vi "Calib_Ch_setup.vi"(1 "Preston tube diammeter in mm":dbl, 2 "Ch & spans":T1(array[cluster])=[{"high limit (10V)"=5.0, "low limit (-10V)"=3.0, "Ch No"=1, "Var name"="Cross wire 1"}, {"high limit (10V)"=5.0, "low limit (-10V)"=3.0, "Ch No"=2, "Var name"="Cross wire 2"}] {"Ch No" min=0 max=7; "low limit (-10V)" min=-10 max=10 format="%.3f"; "high limit (10V)" min=-10 max=10 format="%.3f"}, 3 "Calib filename":path) -> (0 "Output string":string)   [LabVIEW 2010]
panel:
  out "length":i32
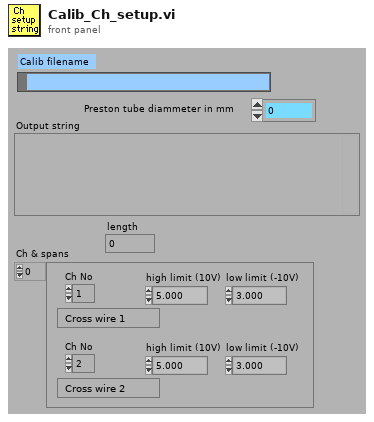
[diagram p1: front panel]
types:
  T1 = cluster{"high limit (10V)":sgl, "low limit (-10V)":sgl, "Ch No":i16, "Var name":string}[]
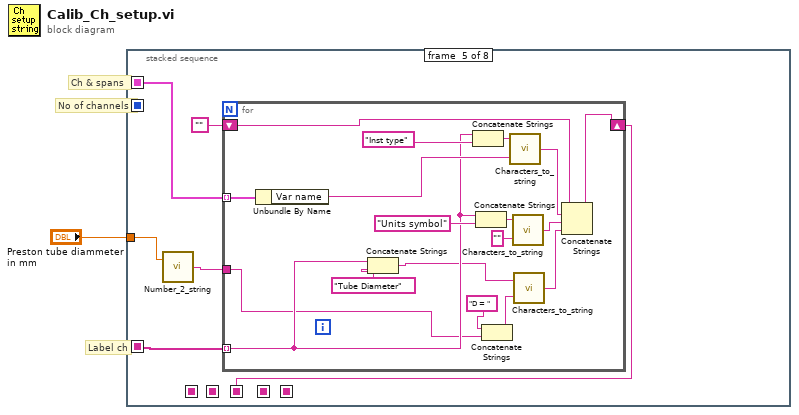
[diagram p0: block diagram]
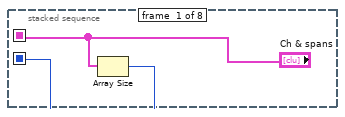
[diagram p2: hidden frame]
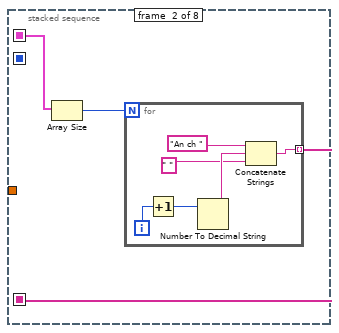
[diagram p3: hidden frame]
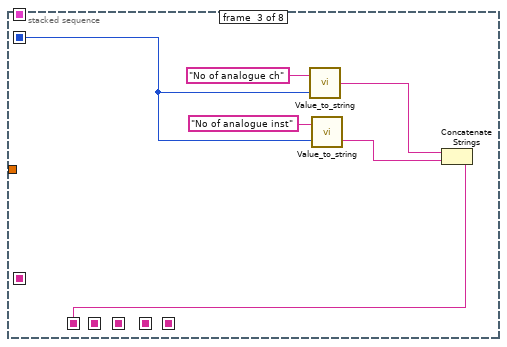
[diagram p4: hidden frame]
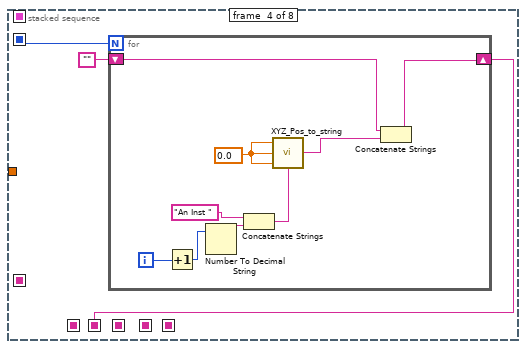
[diagram p5: hidden frame]
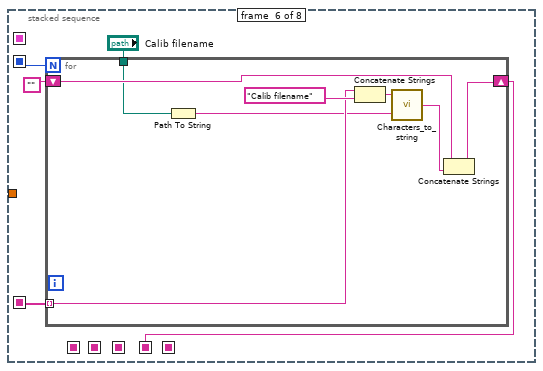
[diagram p6: hidden frame]
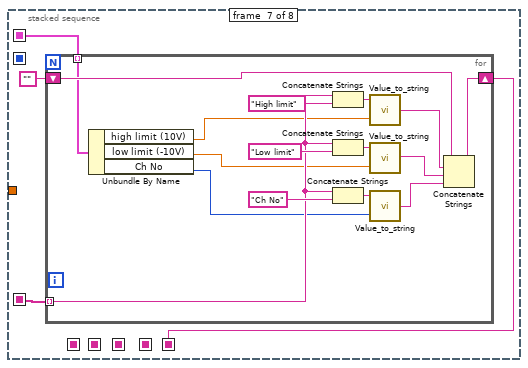
[diagram p7: hidden frame]
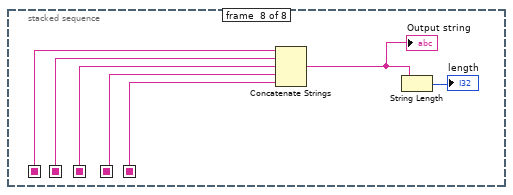
[diagram p8: hidden frame]
diagram:
  # "No of channels"
  # "Ch & spans"
  # "Label ch"
  n1 = stacked-sequence {
    seq-local: [_ _ _ _ w35 _ _ _] -> [_ _ _ _ _ _ _ w94]
    seq-local: [_ _ _ _ _ w57 _ _] -> [_ _ _ _ _ _ _ w93]
    seq-local: [_ _ _ w20 _ _ _ _] -> [_ _ _ _ _ _ _ w92]
    seq-local: [_ w5 _ _ _ _ _ _] -> [_ _ _ _ w34 w58 w70 _]
    seq-local: [_ _ w14 _ _ _ _ _] -> [_ _ _ _ _ _ _ w89]
    seq-local: [_ _ _ _ _ _ w68 _] -> [_ _ _ _ _ _ _ w88]
    seq-local: ["Ch & spans" _ _ _ _ _ _ _] -> [_ w4 _ _ w33 _ w69 _]
    seq-local: [w2 _ _ _ _ _ _ _] -> [_ _ w13 w19 _ w55 _ _]
    tunnel: "Preston tube diammeter in mm" -> [_ _ _ _ w32 _ _ _]
    frame #0 {
      n2 = Array Size(array="Ch & spans") -> (size(s)=w2:i32)
    }
    frame #1 {
      n3 = Array Size(array=w4) -> (size(s)=w6:i32)
      n4 = for {
        N: w6 -> [_]
        tunnel: [w8] -> w5 mode=indexing
        i -> [w10]
        n5 = Increment(x=w10) -> (x+1=w9:i32)
        n6 = Number To Decimal String(number=w9) -> (decimal integer string=w12:string)  [unwired: 1 out]
        n7 = Concatenate Strings("An ch ", w12, " ") -> (w8:string)
      }
    }
    frame #2 {
      n8 = call "Value_to_string.vi"("Value"=w13, "Label for value"="No of analogue ch") -> ("Output string"=w16:string)  [unwired: 1 in]
      n9 = call "Value_to_string.vi"("Value"=w13, "Label for value"="No of analogue inst") -> ("Output string"=w15:string)  [unwired: 1 in]
      n10 = Concatenate Strings(w16, w15) -> (w14:string)
    }
    frame #3 {
      n11 = for {
        N: w19 -> [_]
        shift-right: [w29] -> w20
        shift-left: "" -> [w30]
        i -> [w22]
        w23 = 0.0 ("X")
        n12 = Increment(x=w22) -> (x+1=w28:i32)
        n13 = Number To Decimal String(number=w28) -> (decimal integer string=w27:string)  [unwired: 1 out]
        n14 = Concatenate Strings("An Inst ", w27) -> (w25:string)
        n15 = call "XYZ_Pos_to_string.vi"("Position label"=w25, "Z"=w23, "Y"=w23, "X"=w23) -> ("Output string"=w24:string)
        n16 = Concatenate Strings(w30, w24) -> (w29:string)
      }
    }
    frame #4 {
      n17 = call "Number_2_string.vi"("number"=w32) -> ("String"=w31:string)  [unwired: 1 in]
      n18 = for {
        shift-right: [w53] -> w35
        shift-left: "" -> [w54]
        tunnel: w34 -> [w43] mode=indexing
        tunnel: w33 -> [w45] mode=indexing
        tunnel: w31 -> [w38]
        n19 = Unbundle By Name(w45) -> ("Var name"=w44:string)
        n20 = Concatenate Strings(w43, "Tube Diameter") -> (w41:string)
        n21 = Concatenate Strings(w43, "Inst type") -> (w47:string)
        n22 = Concatenate Strings(w43, "Units symbol") -> (w48:string)
        n23 = Concatenate Strings("D = " ("String to match"), w38) -> (w37:string)
        n24 = call "Characters_to_string.vi"("Characters to write"=w44, "Label for characters"=w47) -> ("Output string"=w49:string)
        n25 = call "Characters_to_string.vi"("Characters to write"="", "Label for characters"=w48) -> ("Output string"=w50:string)
        n26 = call "Characters_to_string.vi"("Characters to write"=w37, "Label for characters"=w41) -> ("Output string"=w40:string)
        n27 = Concatenate Strings(w54, w49, w50, w40) -> (w53:string)
      }
    }
    frame #5 {
      n28 = for {
        N: w55 -> [_]
        shift-right: [w66] -> w57
        shift-left: "" -> [w67]
        tunnel: w58 -> [w62] mode=indexing
        tunnel: "Calib filename" -> [w61]
        n29 = Path To String(path=w61) -> (string=w60:string)
        n30 = Concatenate Strings(w62, "Calib filename") -> (w63:string)
        n31 = call "Characters_to_string.vi"("Characters to write"=w60, "Label for characters"=w63) -> ("Output string"=w64:string)
        n32 = Concatenate Strings(w67, w64) -> (w66:string)
      }
    }
    frame #6 {
      n33 = for {
        shift-right: [w86] -> w68
        shift-left: "" -> [w87]
        tunnel: w70 -> [w76] mode=indexing
        tunnel: w69 -> [w72] mode=indexing
        n34 = Unbundle By Name(w72) -> ("high limit (10V)"=w73:sgl, "low limit (-10V)"=w74:sgl, "Ch No"=w75:i16)
        n35 = Concatenate Strings(w76, "High limit") -> (w83:string)
        n36 = Concatenate Strings(w76, "Low limit") -> (w82:string)
        n37 = Concatenate Strings(w76, "Ch No") -> (w79:string)
        n38 = call "Value_to_string.vi"("Value"=w73, "Label for value"=w83) -> ("Output string"=w84:string)  [unwired: 1 in]
        n39 = call "Value_to_string.vi"("Value"=w74, "Label for value"=w82) -> ("Output string"=w78:string)  [unwired: 1 in]
        n40 = call "Value_to_string.vi"("Value"=w75, "Label for value"=w79) -> ("Output string"=w77:string)  [unwired: 1 in]
        n41 = Concatenate Strings(w87, w84, w78, w77) -> (w86:string)
      }
    }
    frame #7 {
      n42 = Concatenate Strings(w89, w92, w94, w93, w88) -> (w90:string)
      "Output string" <- w90
      n43 = String Length(string=w90) -> (length=→"length":i32)
    }
  }
